vi "Test_ConstructBinding_LatchingBoolean_TypeError.vi"(8 "error in (no error)":errorcluster, 11 "TestCase in":refnum<class "TestTerminalSignalingValueBinding.lvclass">) -> (0 "error out":errorcluster, 3 "TestCase out":refnum<class "TestTerminalSignalingValueBinding.lvclass">)   [LabVIEW 2017, in "TestTerminalSignalingValueBinding.lvclass"]
uses:
  TestTerminalSignalingValueBinding.lvclass
  Source/Concrete/TerminalSignalingValueBinding/TerminalSignalingValueBinding.lvclass
panel:
  out "Return Error":errorcluster
  in  "OK Button":bool
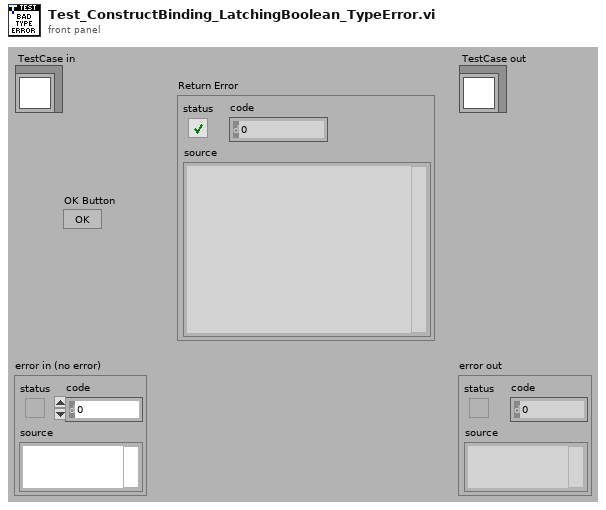
[diagram p1: front panel]
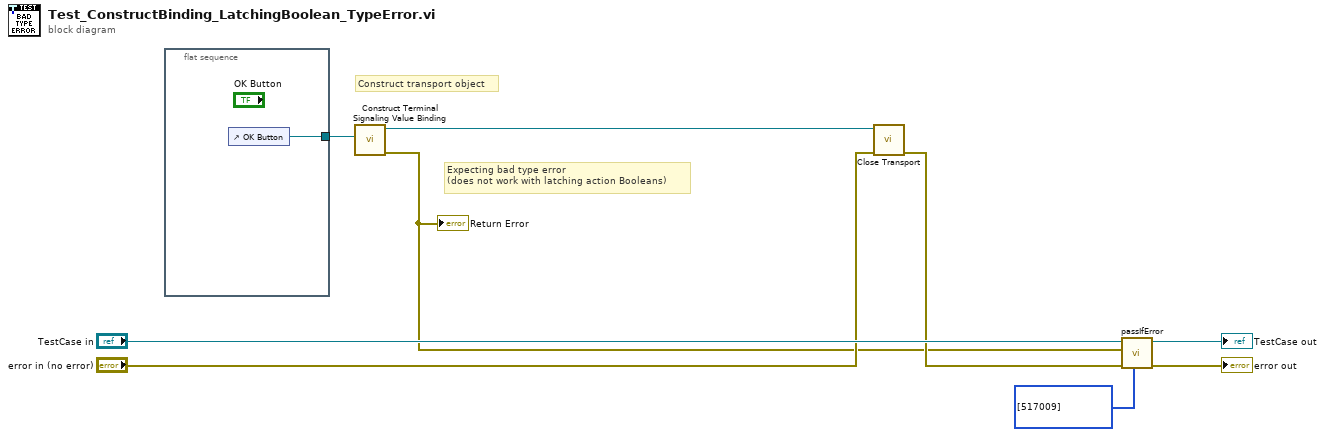
[diagram p0: block diagram]
diagram:
  # "Expecting bad type error\n(does not work with latching action Booleans)"
  # "Construct transport object"
  n1 = flat-sequence {
    tunnel: [w10] -> w5
    frame #0 {
      n2 = control-ref of="OK Button"() -> (w10:refnum<vi>)
    }
  }
  n3 = call "Construct Terminal Signaling Value Binding.vi"("Ctl Refnum"=w5) -> ("error out"=w2:errorcluster, "TerminalSignalingValueBinding"=w6:refnum<class "TerminalSignalingValueBinding.lvclass">)  [unwired: 9 in]
  "Return Error" <- w2
  n4 = call-dynamic "Close Transport.vi"("error in (no error)"="error in (no error)", "ITransport in"=w6) -> ("error out"=w3:errorcluster)  [unwired: 9 in]
  n5 = call-dynamic "passIfError.vi"("passing error codes (default = any error code)"=i32[] [517009], "error in (no error)"=w3, "error"=w2, "TestCase in"="TestCase in") -> ("error out"=→"error out":errorcluster, "TestCase out"=→"TestCase out":refnum<class "TestTerminalSignalingValueBinding.lvclass">)  [unwired: 6 in]
